vi "Realsense Cam Create.vi"(7 "Connect (T)":bool=TRUE, 8 "error in (no error)":errorcluster, 9 "Sensor Index (0)":i32, 10 "Device Index (0)":i32, 11 "Realsense Cam Wrapper in":refnum<class "Realsense Cam Wrapper.lvclass">) -> (0 "error out":errorcluster, 1 "Found?":bool, 2 "init error":string, 3 "Realsense Cam Wrapper out":refnum<class "Realsense Cam Wrapper.lvclass">)   [LabVIEW 2018, in "Realsense Cam Wrapper.lvclass"]
uses:
  Realsense Cam Wrapper.lvclass
  Realsense Cam Wrapper.lvclass/Realsense Cam Wrapper.ctl
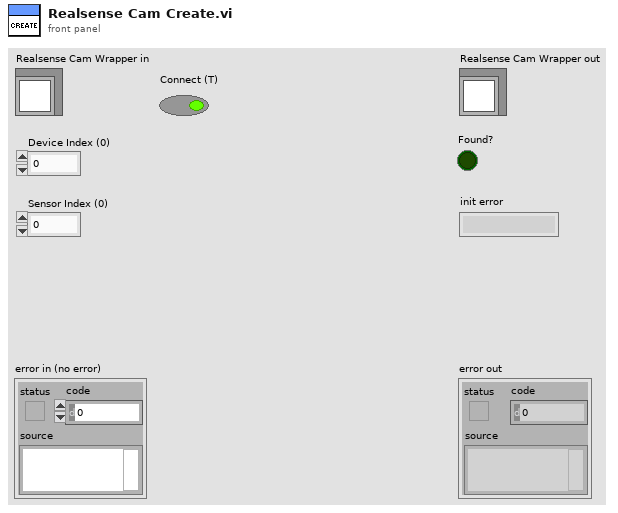
[diagram p1: front panel]
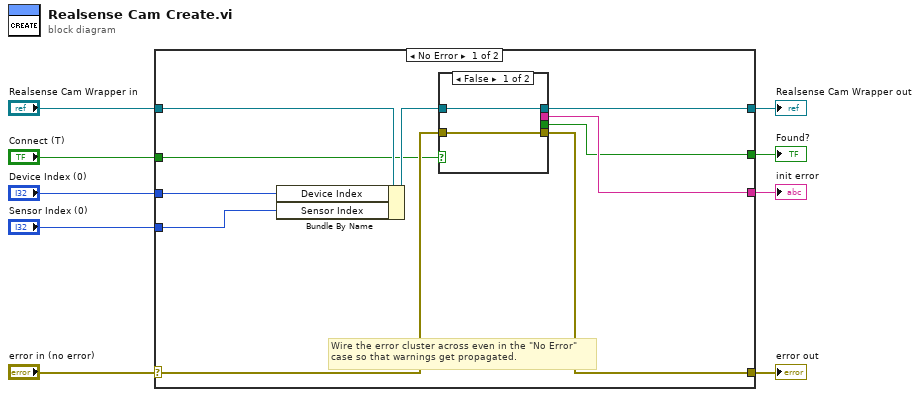
[diagram p0: block diagram]
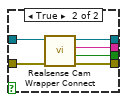
[diagram p2: hidden frame]
diagram:
  n1 = case shown="No Error" "error in (no error)" {
    selector: "error in (no error)" -> [w12 w29]
    tunnel: [w11 w29] -> w8
    tunnel: [w15 w28] -> w6
    tunnel: "Realsense Cam Wrapper in" -> [w19 w28]
    tunnel: "Connect (T)" -> [w10 _]
    tunnel: "Device Index (0)" -> [w18 _]
    tunnel: "Sensor Index (0)" -> [w17 _]
    tunnel: [w14 _] -> w2
    tunnel: [w13 _] -> w1
    frame No Error {
      # "Wire the error cluster across even in the \"No Error\"\ncase so that warnings get propagated."
      n2 = Bundle By Name(cluster=w19, "Device Index"=w18, "Sensor Index"=w17) -> (w16:refnum<class "Realsense Cam Wrapper.lvclass">)
      n3 = case shown="False" w10 {
        tunnel: w16 -> [w21 w27]
        tunnel: [w21 w26] -> w15
        tunnel: [_ w25] -> w14
        tunnel: [_ w24] -> w13
        tunnel: w12 -> [w20 w23]
        tunnel: [w20 w22] -> w11
        frame False {
        }
        frame True {
          n4 = call-dynamic "Realsense Cam Wrapper Connect.vi"("error in (no error)"=w23, "Realsense Cam Wrapper in"=w27) -> ("error out"=w22:errorcluster, "Found?"=w24:bool, "init error"=w25:string, "Realsense Cam Wrapper out"=w26:refnum<class "Realsense Cam Wrapper.lvclass">)  [unwired: 6 in]
        }
      }
    }
    frame Error {
    }
  }
  "error out" <- w8
  "Realsense Cam Wrapper out" <- w6
  "Found?" <- w1
  "init error" <- w2
